vi "configuration.path.vi"() -> (2 "configuration file":path)   [LabVIEW 2020]
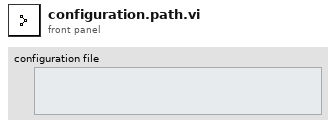
[diagram p1: front panel]
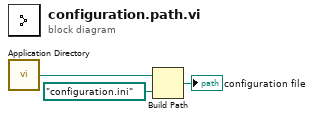
[diagram p0: block diagram]
diagram:
  n1 = call <vilib>:"Application Directory.vi"() -> ("Application Directory"=w1:path)
  n2 = Build Path(base path=w1, name or relative path=path "configuration.ini") -> (appended path=→"configuration file":path)
